vi "classes array.vi"() -> (0 "WSs":refnum<class "WebSocket Client CR.lvclass">[](array[class]))   [LabVIEW 2021, in "WebSockets.lvlib" / "WebSocket Client CR.lvclass"]
uses:
  WebSocket Client CR.lvclass
  WebSocket Client CR.lvclass/WebSocket Client CR.ctl
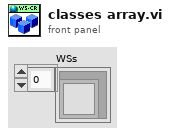
[diagram p1: front panel]
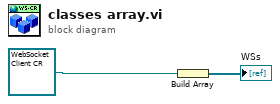
[diagram p0: block diagram]
diagram:
  n1 = Build Array(refnum<class "WebSocket Client CR.lvclass"> refnum ("WebSockets.lvlib:WebSocket Client CR.lvclass")) -> (→"WSs":refnum<class "WebSocket Client CR.lvclass">[])
